vi "Parse CLI Inputs - Application.vi"(8 "error in (no error)":errorcluster, 11 "Arguments":string[](array[string])) -> (0 "error out":errorcluster, 2 "CLI Inputs":T1)   [LabVIEW 2019]
uses:
  CLI Inputs.ctl
  <vilib>/AppBuilder/AB_API/common/AB_API Version Number.ctl
  <vilib>/ErrorRing/Error Ring.xnode
  <vilib>/Utility/error.llb/Error Cluster From Error Code.vi
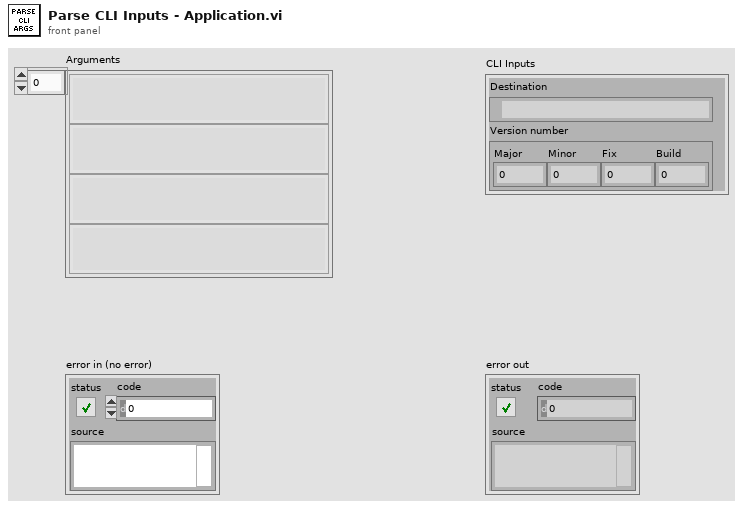
[diagram p1: front panel]
types:
  T1 = typedef "CLI Inputs.ctl" = cluster{"DestDir":path, "Version number":T2}
  T2 = typedef "AB_API Version Number.ctl" = cluster{"Major":u16, "Minor":u16, "Fix":u16, "Build":u16}
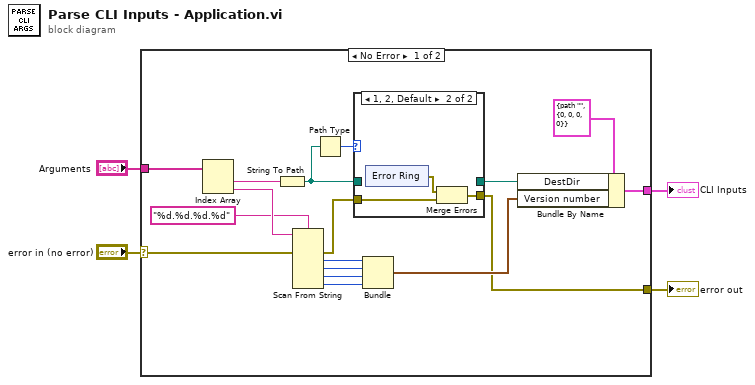
[diagram p0: block diagram]
diagram:
  n1 = case shown="No Error" "error in (no error)" {
    selector: "error in (no error)" -> [w19 w31]
    tunnel: "Arguments" -> [w21 _]
    tunnel: [w12 _] -> w2
    tunnel: [w5 w31] -> w1
    frame No Error {
      n2 = Index Array(array=w21) -> (element #1=w10:string, element #2=w20:string)  [unwired: 2 in]
      n3 = String To Path(string=w10) -> (path=w8:path)
      n4 = Scan From String(format string="%d.%d.%d.%d", input string=w20, error in=w19) -> (error out=w6:errorcluster, output 1=w17:i32, output 2=w16:i32, output 3=w15:i32, output 4=w14:i32)  [unwired: 5 in, 2 out]
      n5 = Path Type(1:w8) -> (0:w9:i16)
      n6 = case shown="1, 2, Default" w9 {
        tunnel: w8 -> [w23 _]
        tunnel: [w23 _] -> w7
        tunnel: w6 -> [w22 w26]
        tunnel: [w22 w24] -> w5
        frame 0 {
        }
        frame 1, 2, Default {
          n7 = xnode "Error Ring"() -> ("error out"=w25:errorcluster)
          n8 = Merge Errors(w25, w26) -> (w24:errorcluster)
        }
      }
      n9 = Bundle(w17, w16, w15, w14) -> (w11:cluster{i32, i32, i32, i32})  [unwired: 1 in]
      n10 = Bundle By Name(cluster=T1 {"DestDir"=path "", "Version number"={"Major"=0, "Minor"=0, "Fix"=0, "Build"=0}} ("CLI Inputs"), "DestDir"=w7, "Version number"=w11) -> (w12:T1)
    }
    frame Error {
    }
  }
  "error out" <- w1
  "CLI Inputs" <- w2
